vi "Level Meter.vi"(8 "error in (no error)":errorcluster, 11 "Level Meter in":refnum<class "Level Meter.lvclass">) -> (0 "error out":errorcluster, 3 "Level Meter out":refnum<class "Level Meter.lvclass">)   [LabVIEW 2017, in "Level Meter.lvclass"]
uses:
  Level Meter.lvclass
  C:/LabVIEW-programs/Instruments/Utility Classes/Readable/Readable.lvclass
  Utility Classes/Readable/Channel Units.ctl
  Utility Classes/Readable/Channel Names.ctl
  Level Meter.lvclass/Level Meter.ctl
  Global/GPIB Numbers.vi
  Utility Classes/Readable/Readable.lvclass
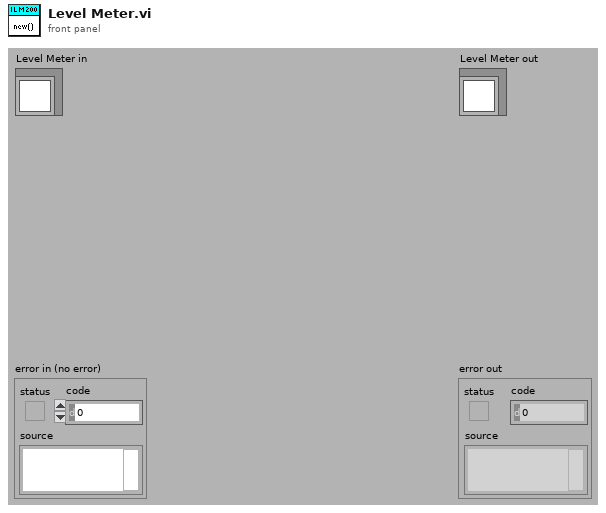
[diagram p1: front panel]
types:
  T1 = typedef "Readable.lvclass/Channel Names.ctl" = string[]
  T2 = typedef "Readable.lvclass/Channel Units.ctl" = string[]
  T3 = typedef "OxfordAddress.ctl" = cluster{"Com Port":i32, "ISOBUS Address":i32, "GPIB Address":i16, "Communication":enum16{"RS232", "ISOBUS", "GPIB", "Gateway"}}
  T4 = cluster{"Address":T3, "ILM Name":string, "Display Channel":i32[]}
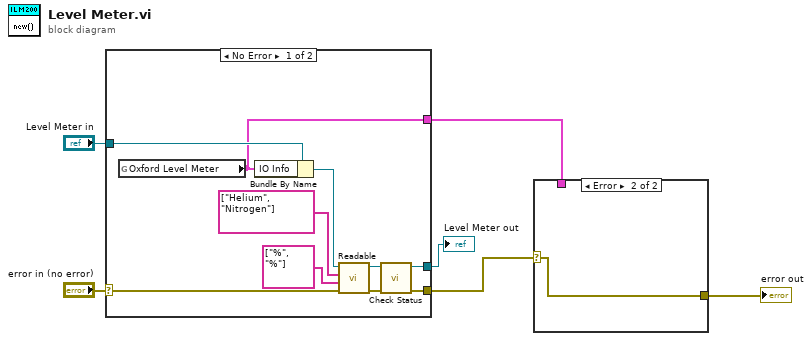
[diagram p0: block diagram]
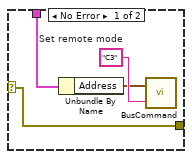
[diagram p2: hidden frame]
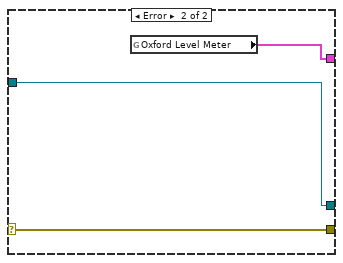
[diagram p3: hidden frame]
diagram:
  n1 = case shown="No Error" "error in (no error)" {
    selector: "error in (no error)" -> [w11 w19]
    tunnel: [w8 w19] -> w3
    tunnel: [w10 w18] -> w4
    tunnel: "Level Meter in" -> [w16 w18]
    tunnel: [w7 w17] -> w1
    frame No Error {
      n2 = global read "GPIB Numbers.vi" "Oxford Level Meter"() -> (w7:T4)
      n3 = Bundle By Name(cluster=w16, "IO Info"=w7) -> (w15:refnum<class "Level Meter.lvclass">)
      n4 = call "Readable.vi"("error in (no error)"=w11, "Channel Units"=T2 ["%", "%"], "Channel Names"=T1 ["Helium", "Nitrogen"], "Readable in"=w15) -> ("error out"=w9:errorcluster, "Readable out"=w14:refnum<class "Level Meter.lvclass">)  [unwired: 6 in]
      n5 = call-dynamic "Check Status.vi"("error in (no error)"=w9, "Level Meter in"=w14) -> ("error out"=w8:errorcluster, "Level Meter out"=w10:refnum<class "Level Meter.lvclass">)  [unwired: 6 in, 2 out]
    }
    frame Error {
      n6 = global read "GPIB Numbers.vi" "Oxford Level Meter"() -> (w17:T4)
    }
  }
  "Level Meter out" <- w4
  n7 = case shown="Error" w3 {
    selector: w3 -> [w23 w24]
    tunnel: [w23 w24] -> w2
    tunnel: w1 -> [w20 _]
    frame No Error {
      w22 = "C3"  # Set remote mode
      n8 = Unbundle By Name(w20) -> ("Address"=w21:T3)
      n9 = call "BusCommand.vi"("Command"=w22, "Instrument address (in)"=w21) -> ()  [unwired: 2 out]
    }
    frame Error {
    }
  }
  "error out" <- w2
